vi "uintArrayMultiplyElements.vi"(8 "Error in (no error)":errorcluster, 11 "Uint array in":refnum<class "UintClass.lvclass">[](array[class])) -> (0 "Error out":errorcluster, 1 "Timing":u32, 3 "Product":refnum<class "UintClass.lvclass">)   [LabVIEW 2011, in "UintClass.lvclass"]
uses:
  UintClass.lvclass
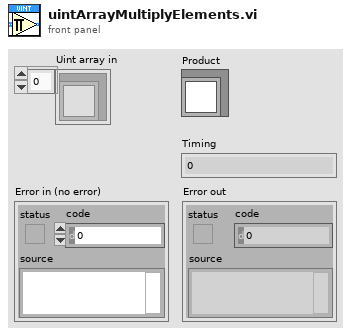
[diagram p1: front panel]
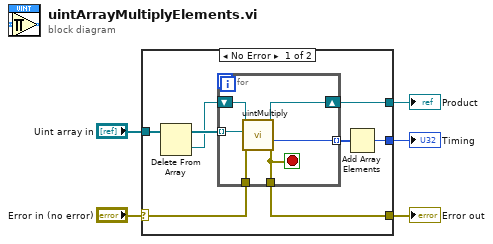
[diagram p0: block diagram]
diagram:
  n1 = case shown="No Error" "Error in (no error)" {
    selector: "Error in (no error)" -> [w13 w20]
    tunnel: "Uint array in" -> [w8 _]
    tunnel: [w12 w20] -> w3
    tunnel: [w11 _] -> w2
    tunnel: [w9 _] -> w1
    frame No Error {
      n2 = Delete From Array(array=w8) -> (deleted portion=w6:refnum<class "UintClass.lvclass">, array with subset deleted=w7:refnum<class "UintClass.lvclass">[])  [unwired: 2 in]
      n3 = for {
        tunnel: w7 -> [w19] mode=indexing
        shift-right: [w18] -> w11
        shift-left: w6 -> [w17]
        tunnel: [w16] -> w10 mode=indexing
        tunnel: w13 -> [w15]
        tunnel: [w14] -> w12
        stop <- w14 stop-if-true
        n4 = call "uintMultiply.vi"("Error in (no error)"=w15, "Uint2 in"=w19, "Uint1 in"=w17) -> ("Error out"=w14:errorcluster, "Timing"=w16:u32, "Uint1 * Uint2"=w18:refnum<class "UintClass.lvclass">)  [unwired: 6 in]
      }
      n5 = Add Array Elements(numeric array=w10) -> (sum=w9:u32)
    }
    frame Error {
    }
  }
  "Error out" <- w3
  "Product" <- w2
  "Timing" <- w1
